vi "NI_9472_DO_Test.vi"() -> ()   [LabVIEW 2014]
uses:
  <vilib>/Platform/TimedLoop/XDataNode/timing_clust.ctl
  <vilib>/Platform/TimedLoop/XDataNode/nitl_modes.ctl
  <vilib>/Platform/TimedLoop/XDataNode/wakeup.ctl
  <vilib>/Platform/TimedLoop/XDataNode/XDataNode.xnode
  <vilib>/Platform/TimedLoop/XDataNode/XDNodeRunTimeDep.lvlib
panel:
  in  "Array":bool[](array[boolean])
  out "error out":errorcluster
  out "mode":i32(ring)=2 items=["Initialization Mode", "Configuration Mode", "Active Mode", "Fault Mode"]
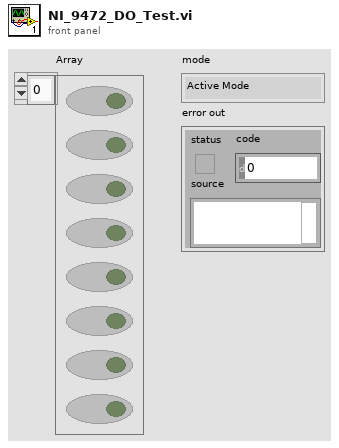
[diagram p1: front panel]
types:
  T1 = typedef "XDNodeRunTimeDep.lvlib/timing_clust.ctl" = cluster{"Expected End [f-1]":u64, "Actual End [f-1]":u64, "Finished Late? [f-1]":bool, "Expected End [i-1]":u64, "Actual End [i-1]":u64, "Finished Late? [i-1]":bool, "Expected Start [i]":u64, "Actual Start [i]":u64, "Expected Start [f]":u64, "Actual Start [f]":u64, "Source Name":string, "Structure Name":string, "Period":i64, "Deadline":i64, "Offset":i64, "Start":i64, "Priority":i32, "Timeout":i32, "Mode":T2, "Wakeup Reason":T3, "Error":errorcluster, "Source Type":string, "Secondary Source Type":string, "Global End Time":u64, "Global Start Time":u64, "Frame Duration":u64, "Iteration Duration":u64, "Assigned CPU":i32, "I/O Scan Engine Mode":u32}
  T2 = typedef "XDNodeRunTimeDep.lvlib/nitl_modes.ctl" = enum32{"No Change", "Process missed periods, maintain original phase", "Discard missed periods, maintain original phase", "Process missed periods, ignore original phase", "Discard missed periods, ignore original phase"}
  T3 = typedef "XDNodeRunTimeDep.lvlib/wakeup.ctl" = enum32{"Normal", "Aborted", "Asynchronous wakeup", "Timing source error", "Timed loop error", "Timeout"}
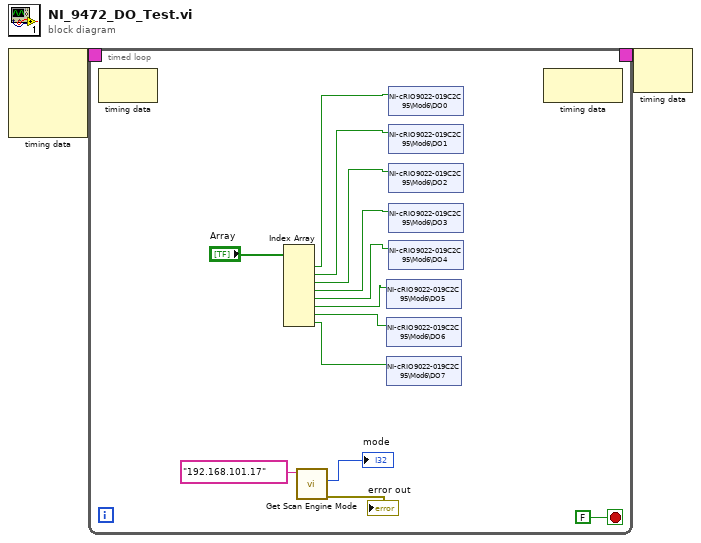
[diagram p0: block diagram]
diagram:
  n1 = node-c288() -> (w2:T1)  [unwired: 4 in]
  n2 = timed-loop {
    timing: w2 -> [_]
    timing-out: [_] -> w1
    stop <- FALSE stop-if-true
    n3 = node-c288() -> ()  [unwired: 1 in, 1 out]
    n4 = Index Array(array="Array") -> (element #1=w10:bool, element #2=w9:bool, element #3=w8:bool, element #4=w7:bool, element #5=w6:bool, element #6=w5:bool, element #7=w4:bool, element #8=w3:bool)  [unwired: 8 in]
    n5 = call <vilib>:"Get Scan Engine Mode.vi"("target address (localhost)"="192.168.101.17") -> ("error out"=→"error out":errorcluster, "mode"=→"mode":i32)  [unwired: 9 in]
    n6 = shared-variable "NI-cRIO9022-019C2C95\\Mod6\\DO5"(w5) -> ()  [unwired: 1 in, 1 out]
    n7 = shared-variable "NI-cRIO9022-019C2C95\\Mod6\\DO6"(w4) -> ()  [unwired: 1 in, 1 out]
    n8 = shared-variable "NI-cRIO9022-019C2C95\\Mod6\\DO7"(w3) -> ()  [unwired: 1 in, 1 out]
    n9 = shared-variable "NI-cRIO9022-019C2C95\\Mod6\\DO0"(w10) -> ()  [unwired: 1 in, 1 out]
    n10 = shared-variable "NI-cRIO9022-019C2C95\\Mod6\\DO1"(w9) -> ()  [unwired: 1 in, 1 out]
    n11 = shared-variable "NI-cRIO9022-019C2C95\\Mod6\\DO2"(w8) -> ()  [unwired: 1 in, 1 out]
    n12 = shared-variable "NI-cRIO9022-019C2C95\\Mod6\\DO3"(w7) -> ()  [unwired: 1 in, 1 out]
    n13 = shared-variable "NI-cRIO9022-019C2C95\\Mod6\\DO4"(w6) -> ()  [unwired: 1 in, 1 out]
    n14 = node-c288() -> ()  [unwired: 1 in, 1 out]
  }
  n15 = node-c288(w1) -> ()  [unwired: 1 out]
